vi "01. Native MQTT Lossy Data Producer.vi"() -> ()   [LabVIEW 2019]
uses:
  <vilib>/ptbypt/NI_PtbyPt.lvlib
panel:
  in  "noise":dbl(slide)=0.2 min=0.0 max=1.0 step=0.1 scale=0.0..1.0
  in  "period (ms)":i32=100 min=5 max=500 step=5
  in  "amplitude":dbl(slide)=2.0 scale=0.0..10.0
  out "Waveform Chart":dbl(graph)
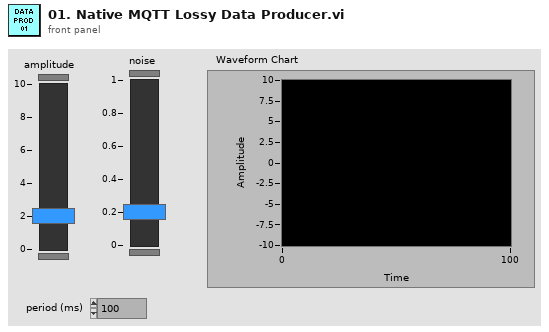
[diagram p1: front panel]
types:
  T1 = typedef "Actor Private Data.ctl" = cluster{"Client":refnum<class "Client.lvclass">, "QualifiedName":string, "EventReg":refnum<event-registration>, "Private Events":T2}
  T2 = typedef "Actor Private Events -- cluster.ctl" = cluster{"Stop":refnum<user-event>, "Subscribe":refnum<user-event>, "Unsubscribe":refnum<user-event>, "publish":refnum<user-event>}
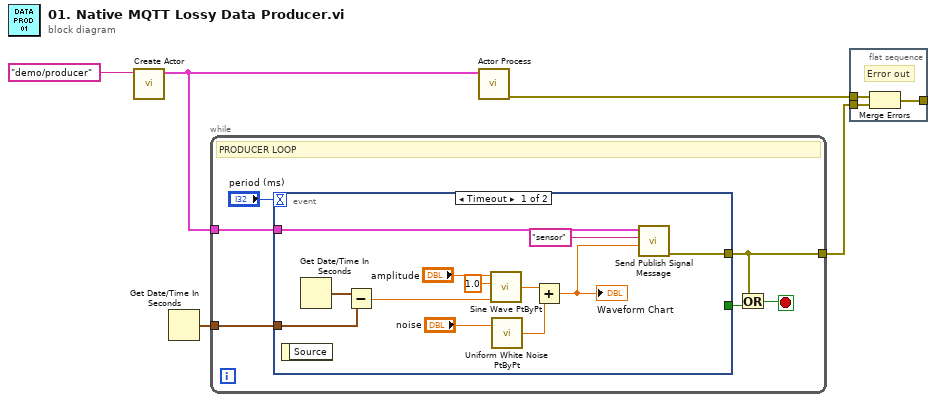
[diagram p0: block diagram]
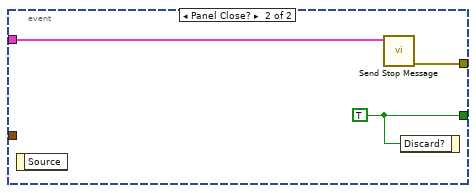
[diagram p2: hidden frame]
diagram:
  n1 = call "Create Actor.vi"("QualifiedName"="demo/producer") -> ("Actor Class"=w4:T1)  [unwired: 9 in, 1 out]
  n2 = Get Date/Time In Seconds() -> (seconds since 1Jan1904=w5:timestamp)
  n3 = while {
    tunnel: w5 -> [w10]
    tunnel: w4 -> [w7]
    tunnel: [w6] -> w1
    stop <- w8 stop-if-true
    # "PRODUCER LOOP"
    n4 = event shown="[0] Timeout" {
      selector: _ -> [_ _]
      dyn-events: _ -> [_ _]
      timeout: "period (ms)" -> [_ _]
      tunnel: w10 -> [w23 _]
      tunnel: [_ w26] -> w9
      tunnel: w7 -> [w14 w25]
      tunnel: [w15 w24] -> w6
      event Timeout {
        n5 = event-data() -> ()  [unwired: 1 in, 1 out]
        n6 = Get Date/Time In Seconds() -> (seconds since 1Jan1904=w16:timestamp)
        n7 = Subtract(x=w16, y=w23) -> (x-y=w17:dbl)
        n8 = call <vilib>:"Sine Wave PtByPt.vi"("time"=w17, "frequency"=1.0, "amplitude"="amplitude") -> ("sine wave"=w21:dbl)  [unwired: 1 in]
        n9 = call <vilib>:"Uniform White Noise PtByPt.vi"("amplitude"="noise") -> ("uniform white noise"=w18:dbl)  [unwired: 2 in]
        n10 = Add(x=w21, y=w18) -> (x+y=w12:dbl)
        "Waveform Chart" <- w12
        n11 = call "Send Publish Signal Message.vi"("Variant"=w12, "Signal Name"="sensor" ("Topic Name (empty: Payload name)"), "Actor Class"=w14) -> ("error out"=w15:errorcluster)  [unwired: 8 in]
      }
      event Panel Close? {
        w26 = TRUE ("Discard?")
        n12 = event-data() -> ()  [unwired: 1 in, 1 out]
        n13 = call "Send Stop Message.vi"("Actor Class"=w25) -> ("error out"=w24:errorcluster)  [unwired: 10 in]
        n14 = event-data("Discard?"=w26) -> ()  [unwired: 1 in, 1 out]
      }
    }
    n15 = Or(x=w6, y=w9) -> (x .or. y?=w8:bool)
  }
  n16 = call "Actor Process.vi"("Actor Class"=w4) -> ("error out"=w2:errorcluster)  [unwired: 10 in]
  n17 = flat-sequence {
    tunnel: w2 -> [w29]
    tunnel: w1 -> [w28]
    tunnel: [w27] -> _
    frame #0 {
      # "Error out"
      n18 = Merge Errors(w29, w28) -> (w27:errorcluster)
    }
  }
